vi "Perform Action.vi"(8 "error in":errorcluster, 10 "Input":variant, 11 "Thermometer DAQmx TC Cont CFG Simulated in":refnum<class "Thermometer DAQmx TC Cont CFG Simulated.lvclass">) -> (0 "error out":errorcluster, 2 "Output":variant, 3 "Thermometer DAQmx TC Cont CFG Simulated out":refnum<class "Thermometer DAQmx TC Cont CFG Simulated.lvclass">)   [LabVIEW 2024, in "DAQmx Simulated CFGs.lvlib" / "Thermometer DAQmx TC Cont CFG Simulated.lvclass"]
uses:
  Thermometer DAQmx TC Cont CFG Simulated.lvclass
  Thermometer DAQmx TC Cont CFG/Thermometer DAQmx TC Cont CFG.lvclass/Thermometer DAQmx TC Cont CFG.ctl
  90a473ef-3655-45e6-a582-1a69a8282fcc.vi
  90a473ef-3655-45e6-a582-1a69a8282fcc.vi/a4169a97-72fc-4003-a778-603cf20cafa0.vi
  <vilib>/JDP Science/JSONtext/Find Item.vi
  <vilib>/JDP Science/JSONtext/Next JSON Value.vi
  <vilib>/JDP Science/JSONtext/String Subset.vi
  <vilib>/JDP Science/JSONtext/Parsing/Advance past next JSON Value (inlined COPY).vi
  <vilib>/JDP Science/JSONtext/Parsing/Advance past whitespace.vi
  <vilib>/JDP Science/JSONtext/Parsing/Advance past String.vi
  <vilib>/JDP Science/JSONtext/Parsing/Advance past Number.vi
  <vilib>/JDP Science/JSONtext/Parsing/Advance past Line Ending.vi
  <vilib>/JDP Science/JSONtext/Parsing/Parse Full Path or Item Name.vi
  <vilib>/JDP Science/JSONtext/Parsing/Advance past Array.vi
  <vilib>/JDP Science/JSONtext/Parsing/Advance past Object.vi
  <vilib>/JDP Science/JSONtext/support/Error Cluster From Code.vi
  <vilib>/JDP Science/JSONtext/Offset/Find Item Locations by Path.vi
  <vilib>/JDP Science/JSONtext/JSON text to Variant.vi
  <vilib>/Utility/error.llb/Error Cluster From Error Code.vi
  <vilib>/JDP Science/JSONtext/LVClass Serializer/JSONtext LVClass Serializer.lvclass
  Thermometer DAQmx TC Cont CFG Simulated.lvclass/Thermometer DAQmx TC Cont CFG Simulated.ctl
  Configurations/CFG JSON/CFG JSON.lvclass
  D:/git/HAL/HAL/Devices/DAQmx/Thermo/Thermometer DAQmx TC Cont CFG/Thermometer DAQmx TC Cont CFG.lvclass
  D:/git/HAL/HAL/Devices/DAQmx/DAQmx Base CFG/DAQmx Base CFG.lvclass
  D:/git/HAL/HAL/Configurations/CFG JSON/CFG JSON.lvclass
  D:/git/HAL/HAL/Configurations/CFG Base/CFG Base.lvclass
  D:/git/HAL/HAL/Devices/DAQmx/Thermo/Thermometer Simulated CFGs/TC Cont CFG/Thermometer DAQmx TC Cont CFG Simulated.lvclass
  Thermometer DAQmx TC Cont CFG/Thermometer DAQmx TC Cont CFG.lvclass
  Buffers/BufferLossless/BufferLossless.lvclass
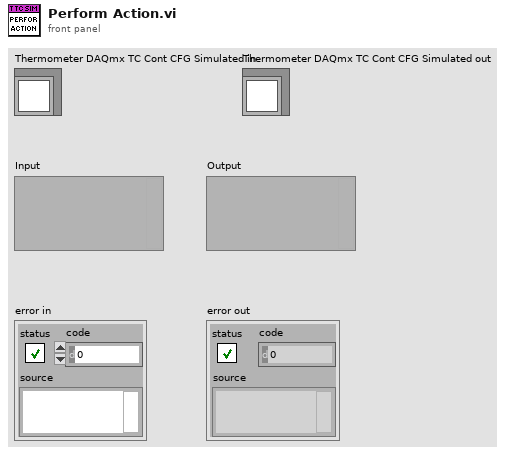
[diagram p1: front panel]
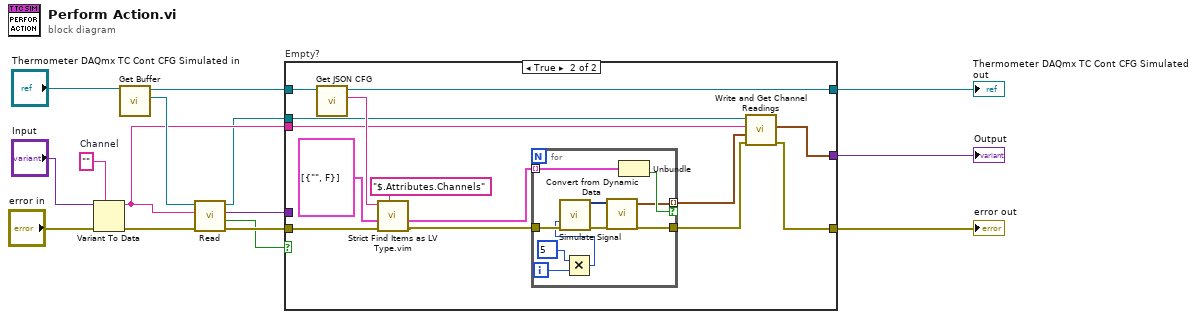
[diagram p0: block diagram]
diagram:
  w11 = ""  # Channel
  n1 = Variant To Data(error in="error in", type=w11, Variant="Input") -> (data=w4:string, error out=w10:errorcluster)
  n2 = call "Get Buffer.vi"("Thermometer DAQmx TC Cont CFG in"="Thermometer DAQmx TC Cont CFG Simulated in") -> ("Buffer Lossless"=w7:refnum<class "BufferLossless.lvclass">, "Thermometer DAQmx TC Cont CFG out"=w6:refnum<class "Thermometer DAQmx TC Cont CFG Simulated.lvclass">)  [unwired: 9 in]
  n3 = call "Read.vi"("error in"=w10, "Channel"=w4, "BufferLossless in"=w7) -> ("error out"=w9:errorcluster, "empty?"=w3:bool, "Readings"=w1:variant, "BufferLossless out"=w2:refnum<class "BufferLossless.lvclass">)  [unwired: 5 in]
  n4 = case "Empty?" shown="True" w3 {
    tunnel: w2 -> [_ w25]
    tunnel: w9 -> [w18 w31]
    tunnel: [w18 w24] -> w15
    tunnel: [w16 w21] -> w14
    tunnel: w4 -> [_ w22]
    tunnel: w6 -> [w17 w28]
    tunnel: [w17 w23] -> w5
    tunnel: w1 -> [w16 _]
    frame False {
    }
    frame True {
      n5 = call "Get JSON CFG.vi"("CFG JSON in"=w28) -> ("<JSON> CFG"=w32:string, "CFG JSON out"=w23:refnum<class "Thermometer DAQmx TC Cont CFG Simulated.lvclass">)  [unwired: 9 in]
      n6 = call "Strict Find Items as LV Type.vim"("$Path or Item Name"="$.Attributes.Channels", "error in"=w31, "Data Type and Default Value"=cluster{"Name":string, "Enabled":bool}[] [{"Name"="", "Enabled"=FALSE}], "<JSON>"=w32) -> ("error out"=w27:errorcluster, "Data out"=w26:cluster{"Name":string, "Enabled":bool}[])  [unwired: 5 in, 1 out]
      n7 = for {
        tunnel: w26 -> [w41] mode=indexing
        tunnel: w27 -> [w40]
        tunnel: [w39] -> w20
        tunnel: [w33] -> w19 mode=indexing if=w35
        i -> [w38]
        n8 = Multiply(x=5, y=w38) -> (x*y=w36:i32)
        n9 = call "Simulate Signal"("Phase"=w36, "error in (no error)"=w40) -> ("Sine with Uniform Noise"=w34:dynamicdata, "error out"=w39:errorcluster)  [unwired: 12 in]
        n10 = call "Convert from Dynamic Data"("Dynamic Data Type"=w34) -> ("Waveform"=w33:waveform(dbl))  [unwired: 3 in]
        n11 = Unbundle(w41) -> ("Enabled"=w35:bool)  [unwired: 1 out]
      }
      n12 = call "Write and Get Channel Readings.vi"("error in"=w20, "Readings"=w19, "Channel"=w22, "BufferLossless in"=w25) -> ("error out"=w24:errorcluster, "Reading"=w21:waveform(dbl))  [unwired: 5 in, 1 out]
    }
  }
  "error out" <- w15
  "Thermometer DAQmx TC Cont CFG Simulated out" <- w5
  "Output" <- w14
